vi "DecodeLookupService.vi"(2 "error in (no error)":errorcluster, 3 "Response":string) -> (0 "error out":errorcluster, 1 "Reply 2":T1(array[cluster]))   [LabVIEW 2010]
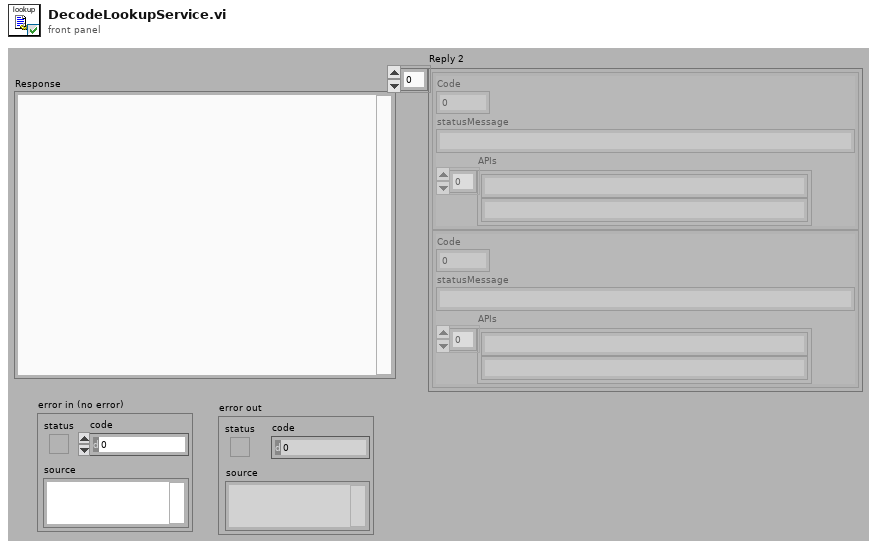
[diagram p1: front panel]
types:
  T1 = cluster{"Code":i8, "statusMessage":string, "APIs":string[]}[]
  T2 = cluster{"Code":i8, "statusMessage":string, "APIs":string[]}
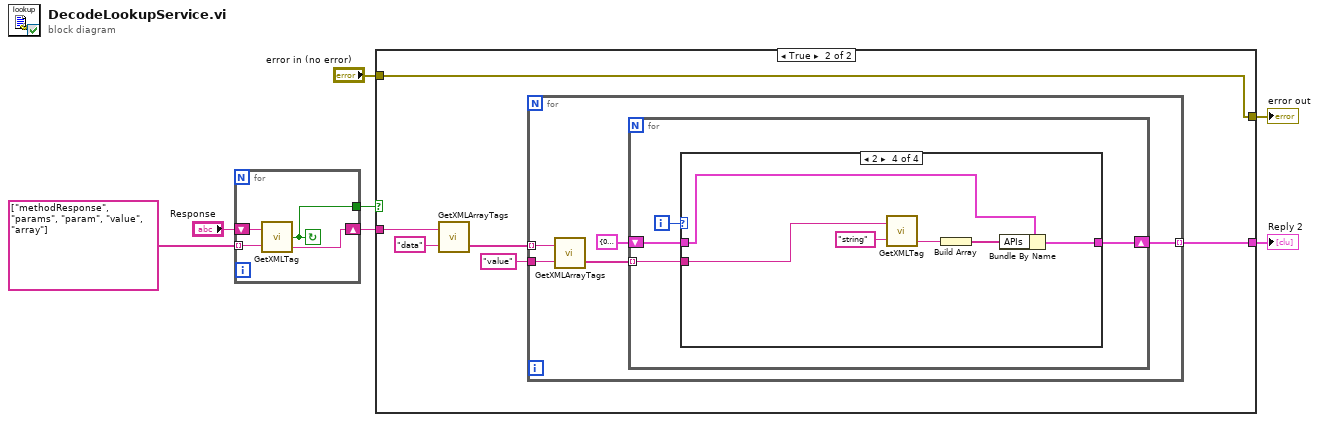
[diagram p0: block diagram]
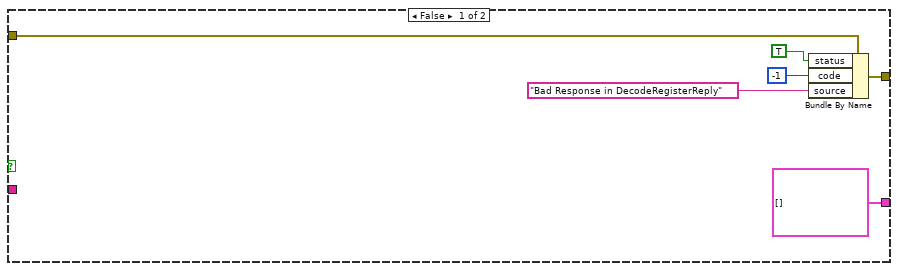
[diagram p2: hidden frame]
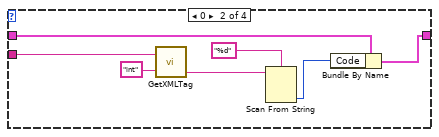
[diagram p4: hidden frame]
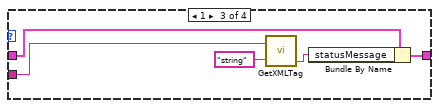
[diagram p5: hidden frame]
diagram:
  n1 = for {
    tunnel: string[] ["methodResponse", "params", "param", "value", "array"] -> [w11] mode=indexing
    shift-right: [w9] -> w6
    shift-left: "Response" -> [w10]
    tunnel: [w8] -> w4
    stop <- w8 continue-if-true
    n2 = call "GetXMLTag.vi"("Tag"=w11, "String"=w10) -> ("Value"=w9:string, "Exists?"=w8:bool)  [unwired: 1 out]
  }
  n3 = case shown="True" w4 {
    tunnel: w6 -> [_ w20]
    tunnel: [T1 [] w19] -> w5
    tunnel: "error in (no error)" -> [w16 w18]
    tunnel: [w15 w18] -> w2
    frame False {
      n4 = Bundle By Name(cluster=w16, "status"=TRUE, "code"=-1, "source"="Bad Response in DecodeRegisterReply") -> (w15:errorcluster)
    }
    frame True {
      n5 = call "GetXMLArrayTags.vi"("ArrayTag"="data", "String"=w20) -> ("Array"=w22:string[])  [unwired: 1 out]
      n6 = for {
        tunnel: w22 -> [w28] mode=indexing
        tunnel: "value" -> [w27]
        tunnel: [w24] -> w19 mode=indexing
        n7 = call "GetXMLArrayTags.vi"("ArrayTag"=w27, "String"=w28) -> ("Array"=w26:string[])  [unwired: 1 out]
        n8 = for {
          tunnel: w26 -> [w32] mode=indexing
          shift-right: [w29] -> w24
          shift-left: T2 {"Code"=0, "statusMessage"="", "APIs"=[]} ("Parameters") -> [w30]
          i -> [w31]
          n9 = case shown="2" w31 {
            tunnel: w32 -> [_ w39 w44 w48]
            tunnel: w30 -> [w33 w36 w43 w51]
            tunnel: [w33 w34 w42 w50] -> w29
            frame Default {
            }
            frame 0 {
              n10 = call "GetXMLTag.vi"("Tag"="int", "String"=w39) -> ("Value"=w38:string)  [unwired: 2 out]
              n11 = Scan From String(format string="%d", input string=w38) -> (output 1=w35:i32)  [unwired: 3 in, 3 out]
              n12 = Bundle By Name(cluster=w36, "Code"=w35) -> (w34:T2)
            }
            frame 1 {
              n13 = call "GetXMLTag.vi"("Tag"="string", "String"=w44) -> ("Value"=w41:string)  [unwired: 2 out]
              n14 = Bundle By Name(cluster=w43, "statusMessage"=w41) -> (w42:T2)
            }
            frame 2 {
              n15 = call "GetXMLTag.vi"("Tag"="string", "String"=w48) -> ("Value"=w47:string)  [unwired: 2 out]
              n16 = Build Array(w47) -> (w46:string[])
              n17 = Bundle By Name(cluster=w51, "APIs"=w46) -> (w50:T2)
            }
          }
        }
      }
    }
  }
  "Reply 2" <- w5
  "error out" <- w2
